vi "SV Stationary Loudness (Time) (1 Ch).vi"(0 "sound pressure signal [Pa]":waveform(dbl)={"t0"=timestamp(0 s since 1904-01-01), "dt"=1.953125e-05, "Y"=[]}, 1 "diffuse field":bool, 2 "restart averaging (F)":bool, 11 "error in (no error)":errorcluster) -> (4 "specific loudness":cluster{dbl[], "Nm":dbl[]}(graph), 6 "loudness [Sone]":dbl format="%.2f", 8 "loudness level [Phon]":dbl format="%.2f", 10 "loudness info":T1, 15 "error out":errorcluster)   [LabVIEW 2017, in "SoundVib_SoundQuality.lvlib"]
doc: "Computes stationary loudness from the sound pressure signal waveform or the 1/3-octave band spectrum calculated over the frequency range 25 Hz to 12.5 kHz. Wire data to the <B>sound pressure signal [Pa]</B> input to determine the polymorphic instance to use or manually select the instance."
uses:
  <vilib>/addons/Sound and Vibration/svt_Sound Quality/SoundVib_SoundQuality.lvlib
  <vilib>/addons/_NISVFA/_Shared subVIs/Controls/svc_SQ Info.ctl
  <vilib>/addons/_NISVFA/_Shared subVIs/Common/SVL Set dB Reference (1 Ch).vi
  <vilib>/addons/_NISVFA/_Shared subVIs/Common/SVL Set dB Reference (variant).vi
  <vilib>/addons/Sound and Vibration/svt_Octave/SVT Third-octave Analysis (1 Ch).vi
  <vilib>/addons/_NISVFA/_Shared subVIs/Common/svc_Caller VI Returned in Error Source.vi
  <vilib>/addons/Sound and Vibration/svt_Octave/SoundVib_Octave.lvlib
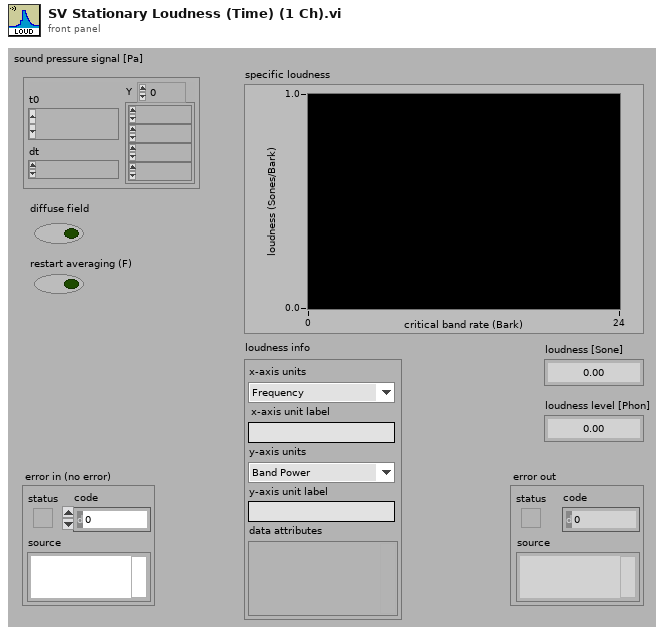
[diagram p1: front panel]
types:
  T1 = typedef "svc_SQ Info.ctl" = cluster{"x-axis units":enum16{"Frequency", "Critical Band", "Critical Band Rate"}, "x-axis unit label":string, "y-axis units":enum16{"Band Power", "Level", "Loudness", "Sharpness", "Roughness", "Fluctuation Strength", "Tonality"}, "y-axis unit label":string, "data attributes":variant}
  T2 = enum16{"Linear", "Exponential", "Equal confidence", "Peak"}
  T3 = cluster{"low band":enum16{"20 Hz", "25 Hz", "31.5 Hz", "40 Hz", "50 Hz", "63 Hz", "80 Hz", "100 Hz", "125 Hz", "160 Hz", "200 Hz", "250 Hz", "315 Hz", "400 Hz", "500 Hz", "630 Hz", "800 Hz", "1000 Hz", "1250 Hz", "1600 Hz", "2000 Hz", "2500 Hz", "3150 Hz", "4000 Hz", "5000 Hz", "6300 Hz", "8000 Hz", "10000 Hz", "12500 Hz", "16000 Hz", "20000 Hz"}, "high band":enum16{"20 Hz", "25 Hz", "31.5 Hz", "40 Hz", "50 Hz", "63 Hz", "80 Hz", "100 Hz", "125 Hz", "160 Hz", "200 Hz", "250 Hz", "315 Hz", "400 Hz", "500 Hz", "630 Hz", "800 Hz", "1000 Hz", "1250 Hz", "1600 Hz", "2000 Hz", "2500 Hz", "3150 Hz", "4000 Hz", "5000 Hz", "6300 Hz", "8000 Hz", "10000 Hz", "12500 Hz", "16000 Hz", "20000 Hz"}}
  T4 = cluster{"nominal frequencies [Hz]":dbl[], "band power":dbl[]}
  T5 = typedef "SoundVib_Octave.lvlib/sv_Octave Info.ctl" = cluster{"standard":T6, "bandwidth":enum16{"1 octave", "1/3 octave", "1/6 octave", "1/12 octave", "1/24 octave"}, "low band":i32, "high band":i32, "weighting filter":T7, "dB reference":dbl, "dB On":bool, "unit label":string, "channel name":string, "description":string, "engineering units":T8, "custom label":string, "spectrum type":enum16{"power", "magnitude"}, "spectral density":bool, "filters settled":bool}
  T6 = typedef "svc_Octave Standard.ctl" = enum16{"ANSI S1.11", "IEC 61260"}
  T7 = typedef "svc_Weighting Filter Text Ring.ctl" = u16
  T8 = typedef "svc_Engineering Units Text Ring.ctl" = u16
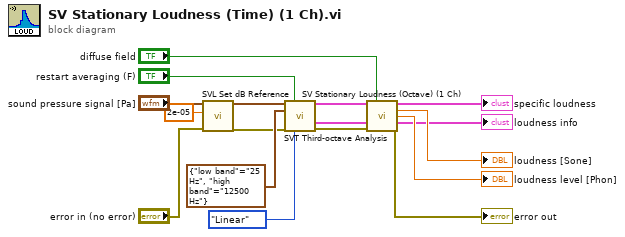
[diagram p0: block diagram]
diagram:
  n1 = call-poly <vilib>:"SVL Set dB Reference.vi"("error in (no error)"="error in (no error)", "dB reference [EU]"=2e-05, "scaled signal in [EU]"="sound pressure signal [Pa]") -> ("error out"=w3:errorcluster, "scaled signal out [EU]"=w5:waveform(dbl))  [unwired: 7 in]
  n2 = call-poly <vilib>:"SVT Third-octave Analysis.vi"("scaled signal [EU]"=w5, "restart averaging (F)"="restart averaging (F)", "frequency range"=T3 {"low band"=enum."25 Hz", "high band"=enum."12500 Hz"}, "error in (no error)"=w3, "averaging type"=T2."Linear") -> ("octave spectrum"=w15:T4, "octave info"=w14:T5, "error out"=w13:errorcluster)  [unwired: 5 in, 3 out]
  n3 = call <vilib>:"SV Stationary Loudness (Octave) (1 Ch).vi"("octave spectrum"=w15, "diffuse field"="diffuse field", "octave info"=w14, "error in (no error)"=w13) -> ("specific loudness"=→"specific loudness":cluster{dbl[], "Nm":dbl[]}, "loudness [Sone]"=→"loudness [Sone]":dbl, "loudness level [Phon]"=→"loudness level [Phon]":dbl, "loudness info"=→"loudness info":T1, "error out"=→"error out":errorcluster)  [unwired: 7 in]
